vi "testKM2.vi"() -> ()   [LabVIEW 2014]
panel:
  out "distancia 2":dbl
  out "m/s":dbl
  out "km/h":dbl
  in  "factor":dbl
  out "error out":errorcluster
  in  "start":bool
  in  "reset":bool
  out "labelTestTime":string caption="Tempo total de ensaio"
  in  "count 2":dbl
  in  "count":dbl
  in  "Distancia":dbl
  out "Frequencia":dbl
  out "Sine":dynamicdata(graph)
  in  "stop":bool
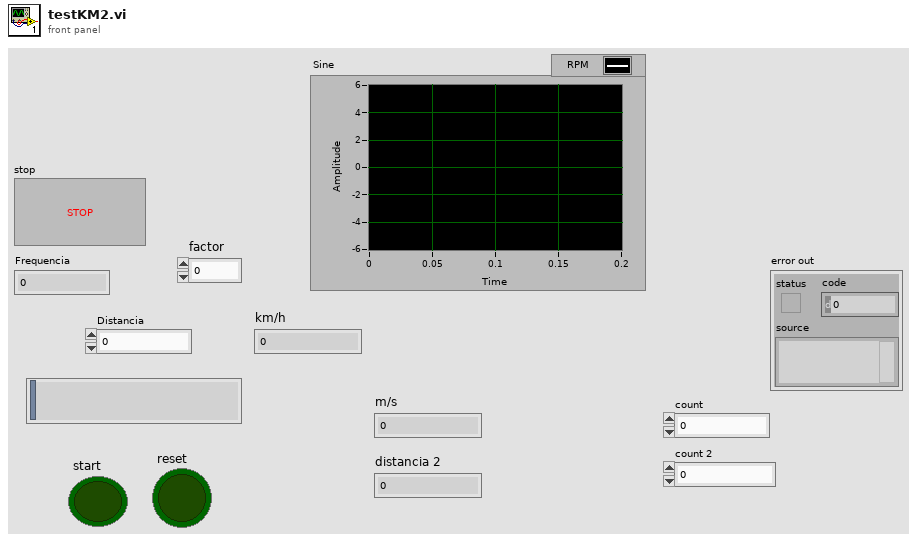
[diagram p1: front panel]
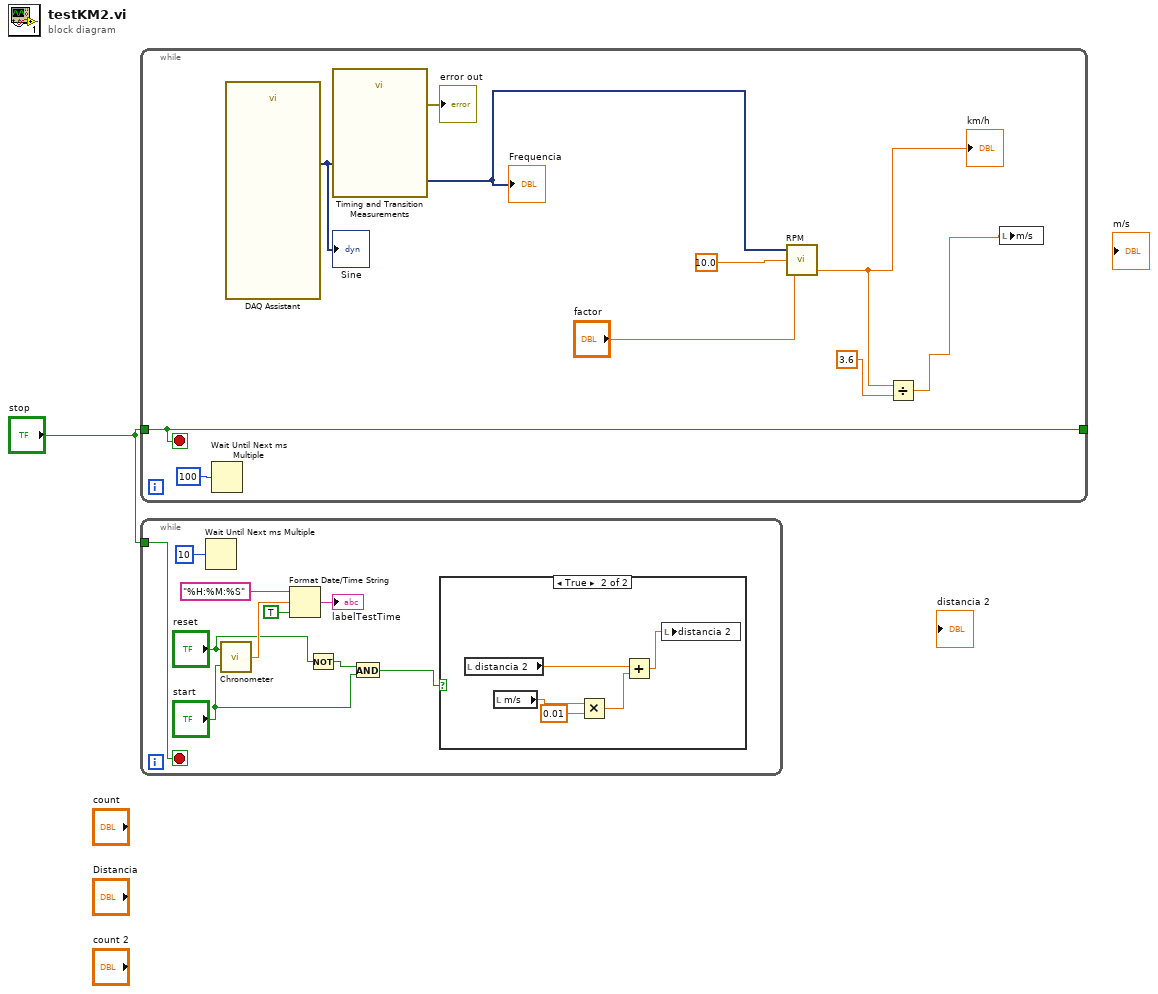
[diagram p0: block diagram]
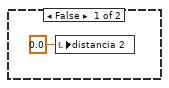
[diagram p2: hidden frame]
diagram:
  n1 = while {
    tunnel: [w9] -> _
    tunnel: "stop" -> [w9]
    stop <- w9 stop-if-true
    n2 = Wait Until Next ms Multiple(millisecond multiple=u32 100) -> ()  [unwired: 1 out]
    n3 = call "DAQ Assistant"() -> ("data"=w10:dynamicdata)  [unwired: 16 in, 3 out]
    "Sine" <- w10
    n4 = call "Timing and Transition Measurements"("Signals"=w10) -> ("error out"=→"error out":errorcluster, "Frequency"=w5:dynamicdata)  [unwired: 9 in]
    "Frequencia" <- w5
    n5 = call "RPM.vi"("factor"="factor", "Lower level"=10.0, "data"=w5) -> ("km/h"=w4:dbl)  [unwired: 2 out]
    "km/h" <- w4
    n6 = Divide(x=w4, y=3.6) -> (x/y=w2:dbl)
    n7 = local write "m/s"(w2) -> ()
  }
  n8 = while {
    tunnel: "stop" -> [w16]
    stop <- w16 stop-if-true
    n9 = Wait Until Next ms Multiple(millisecond multiple=u32 10) -> ()  [unwired: 1 out]
    n10 = call "Chronometer.vi"("start"="start", "reset"="reset") -> ("Time"=w17:dbl)
    n11 = Format Date/Time String(time format string (%c)="%H:%M:%S", seconds (now)=w17, UTC format=TRUE) -> (date/time string=→"labelTestTime":string)
    n12 = Not(x="reset") -> (.not. x?=w15:bool)
    n13 = And(x=w15, y="start") -> (x .and. y?=w12:bool)
    n14 = case shown="True" w12 {
      frame False {
        n15 = local write "distancia 2"(0.0 ("distancia 2")) -> ()
      }
      frame True {
        n16 = local read "distancia 2"() -> (w27:dbl)
        n17 = local read "m/s"() -> (w25:dbl)
        n18 = Multiply(x=w25, y=0.01) -> (x*y=w26:dbl)
        n19 = Add(x=w27, y=w26) -> (x+y=w23:dbl)
        n20 = local write "distancia 2"(w23) -> ()
      }
    }
  }
